vi "HGF_DSCService.appendData2Variant.vi"(0 "initData":variant, 2 "Shared Variable":refnum<k21>, 3 "defaultData":variant, 4 "typeDescriptor":string, 5 "error in (no error)":errorcluster) -> (14 "dup initData":variant, 19 "error out":errorcluster)   [LabVIEW 2012, in "HGF_DSC.lvlib" / "HGF_DSCService.lvclass"]
uses:
  HGF_DSCService.lvclass
panel:
  in  "defaultQuality":i32
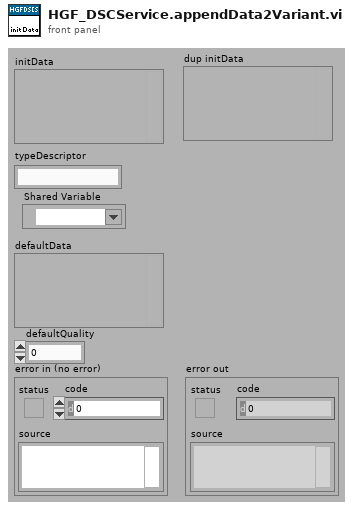
[diagram p1: front panel]
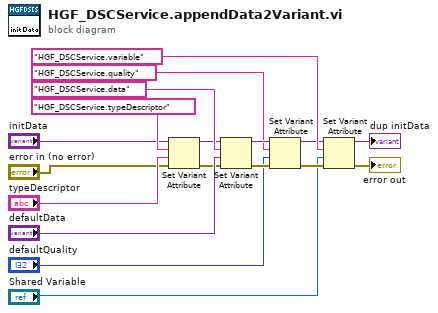
[diagram p0: block diagram]
diagram:
  n1 = Set Variant Attribute(Variant="initData", name="HGF_DSCService.typeDescriptor", value="typeDescriptor", error in="error in (no error)") -> (Variant out=w9:variant, error out=w8:errorcluster)  [unwired: 1 out]
  n2 = Set Variant Attribute(Variant=w9, name="HGF_DSCService.data", value="defaultData", error in=w8) -> (Variant out=w12:variant, error out=w13:errorcluster)  [unwired: 1 out]
  n3 = Set Variant Attribute(Variant=w12, name="HGF_DSCService.quality", value="defaultQuality", error in=w13) -> (Variant out=w15:variant, error out=w16:errorcluster)  [unwired: 1 out]
  n4 = Set Variant Attribute(Variant=w15, name="HGF_DSCService.variable", value="Shared Variable", error in=w16) -> (Variant out=→"dup initData":variant, error out=→"error out":errorcluster)  [unwired: 1 out]
